vi "(SUBTASK 3) - Read and display material.vi"() -> ()   [LabVIEW 2016, in "testrobot.lvrbt"]
uses:
  testrobot.lvrbt
  <vilib>/NXT/Block Support/NXT_InputPort.ctl
  <vilib>/NXT/Subs/LVHSConnector.ctl
  <vilib>/NXT/LegoClasses/BrickReference/BrickReference.lvclass
panel:
  out "Numeric":dbl
  in  "left light":T1 items=["Port 1", "Port 2", "Port 3", "Port 4"]
  in  "right light":T1=3 items=["Port 1", "Port 2", "Port 3", "Port 4"]
  out "only right":bool
  out "both negative":bool
  out "both positve":bool
  out "Left":bool
  out "Right":bool
  out "Right 2":sgl
  out "Left 2":sgl
  out "NXT/EV3 2":T2
  out "Scaled dif":dbl
  in  "NXT/EV3":T2
  in  "Force":T1=1 items=["Port 1", "Port 2", "Port 3", "Port 4"]
  # "Port 2"
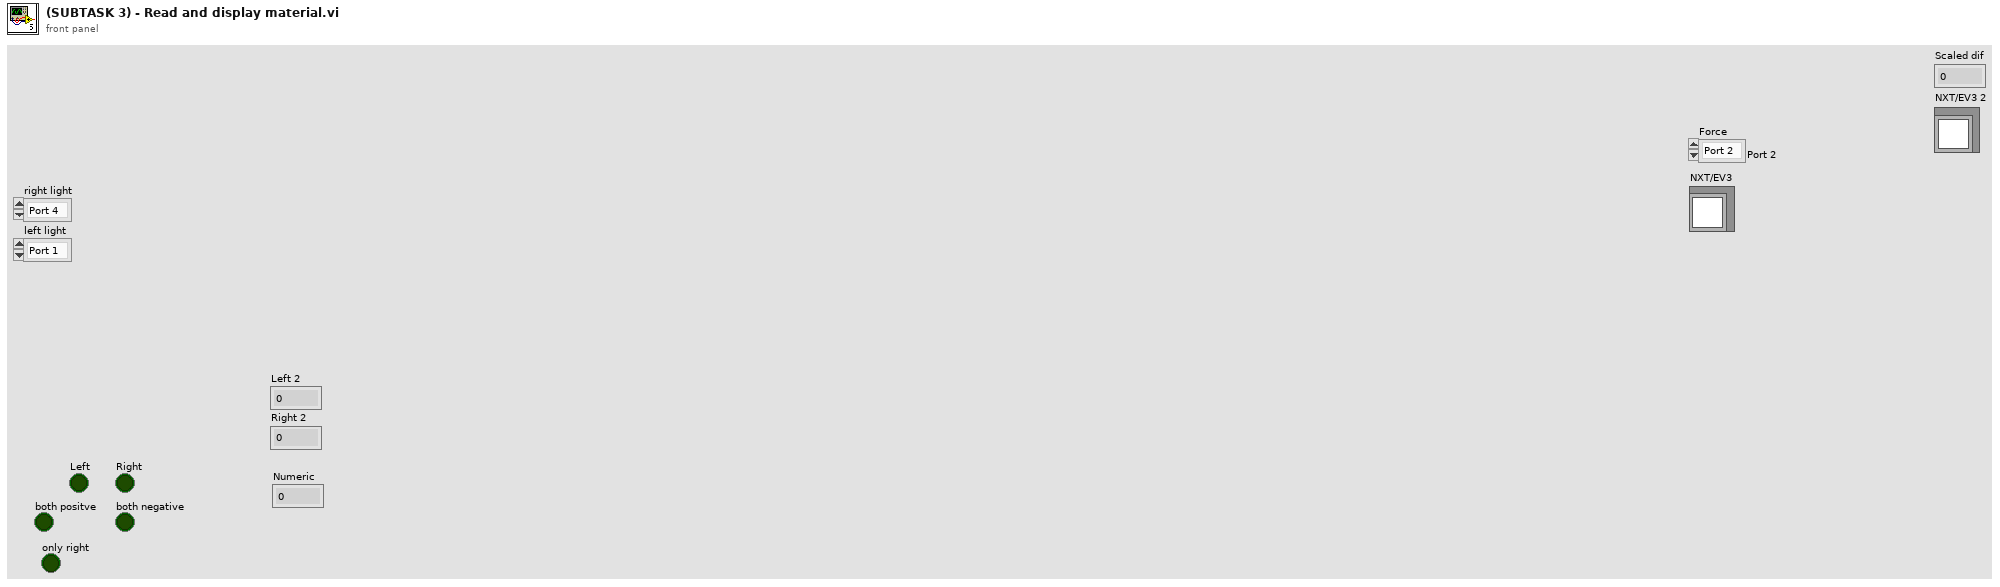
[diagram p1: front panel]
types:
  T1 = typedef "NXT_InputPort.ctl" = u32
  T2 = typedef "LVHSConnector.ctl" = refnum<class "BrickReference.lvclass">
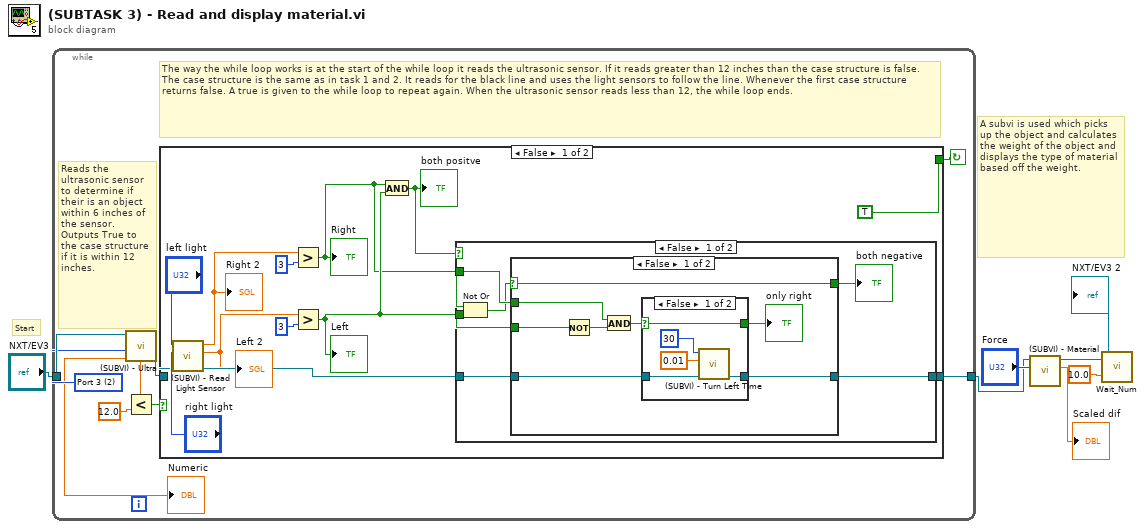
[diagram p0: block diagram]
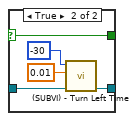
[diagram p2: hidden frame]
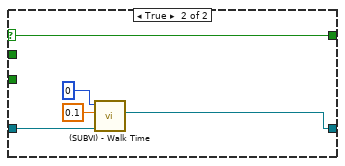
[diagram p3: hidden frame]
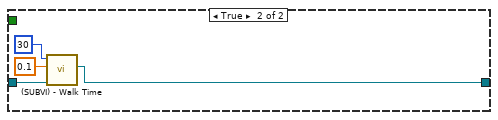
[diagram p4: hidden frame]
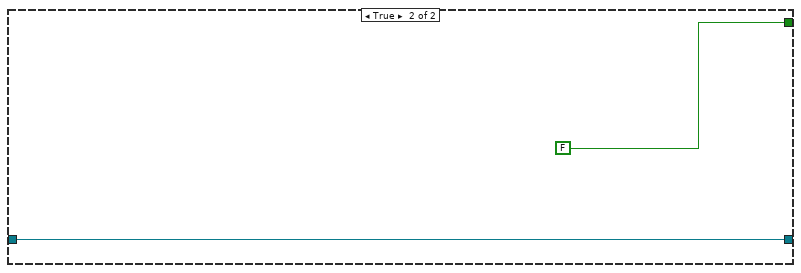
[diagram p5: hidden frame]
diagram:
  # "A subvi is used which picks up the object and calculates the weight of the object and displays the type of material based off the weight."
  # "Start"
  n1 = while {
    tunnel: "NXT/EV3" -> [w15]
    tunnel: [w10] -> w1
    stop <- w12 continue-if-true
    w9 = T1 2 items=["Port 1", "Port 2", "Port 3", "Port 4"] ("Port (Port 1)")
    # "The way the while loop works is at the start of the while loop it reads the ultrasonic sensor. If it reads greater than 12 inches than the case structure is false. The case structure is the same as in task 1 and 2. It reads for the black line and uses the light sensors to follow the line. Whenever the first case structure returns false. A true is given to the while loop to repeat again. When the ultrasonic sensor reads less than 12, the while loop ends."
    # "Reads the ultrasonic sensor to determine if their is an object within 6 inches of the sensor. Outputs True to the case structure if it is within 12 inches."
    n2 = call "(SUBVI) - Ultra.vi"("Port (Port 1)"=w9, "NXT/EV3"=w15) -> ("Inches"=w8:sgl, "NXT/EV3 2"=w11:T2)  [unwired: 8 in]
    "Numeric" <- w8
    n3 = Less?(x=w8, y=sgl 12.0 ("x")) -> (x < y?=w13:bool)
    n4 = case shown="False" w13 {
      tunnel: [TRUE FALSE] -> w12
      tunnel: w11 -> [w18 w62]
      tunnel: [w17 w62] -> w10
      frame False {
        n5 = call "(SUBVI) - Read Light Sensor.vi"("NXT/EV3"=w18, "Port (Port 1) 2"="right light", "Port (Port 1)"="left light") -> ("NXT/EV3 2"=w24:T2, "Scaled Value 2"=w21:sgl, "Scaled Value"=w22:sgl)  [unwired: 6 in]
        "Left 2" <- w21
        "Right 2" <- w22
        n6 = Greater?(x=w22, y=3) -> (0:w25:bool)
        "Right" <- w25
        n7 = Greater?(x=w21, y=3) -> (0:w26:bool)
        "Left" <- w26
        n8 = And(x=w25, y=w26) -> (x .and. y?=w23:bool)
        "both positve" <- w23
        n9 = case shown="False" w23 {
          tunnel: w24 -> [w30 w59]
          tunnel: [w29 w58] -> w17
          tunnel: w25 -> [w33 _]
          tunnel: w26 -> [w32 _]
          frame False {
            n10 = Not Or(1:w32, 2:w33) -> (0:w31:bool)
            n11 = case shown="False" w31 {
              selector: w31 -> [w42 w57]
              tunnel: [w42 w57] -> w34
              tunnel: w33 -> [w40 _]
              tunnel: w32 -> [w38 _]
              tunnel: w30 -> [w36 w54]
              tunnel: [w35 w53] -> w29
              frame False {
                n12 = Not(x=w38) -> (.not. x?=w39:bool)
                n13 = And(x=w40, y=w39) -> (x .and. y?=w41:bool)
                n14 = case shown="False" w41 {
                  selector: w41 -> [w47 w52]
                  tunnel: [w47 w52] -> w37
                  tunnel: w36 -> [w44 w49]
                  tunnel: [w43 w48] -> w35
                  frame False {
                    n15 = call "(SUBVI) - Turn Left Time.vi"("NXT/EV3"=w44, "Time walking"=0.01, "Walk Speed"=30) -> ("NXT/EV3 2"=w43:T2)  [unwired: 8 in]
                  }
                  frame True {
                    n16 = call "(SUBVI) - Turn Left Time.vi"("NXT/EV3"=w49, "Time walking"=0.01, "Walk Speed"=-30) -> ("NXT/EV3 2"=w48:T2)  [unwired: 8 in]
                  }
                }
                "only right" <- w37
              }
              frame True {
                n17 = call "(SUBVI) - Walk Time.vi"("NXT/EV3"=w54, "Time walking"=0.1, "Walk Speed"=0) -> ("NXT/EV3 2"=w53:T2)  [unwired: 8 in]
              }
            }
            "both negative" <- w34
          }
          frame True {
            n18 = call "(SUBVI) - Walk Time.vi"("NXT/EV3"=w59, "Time walking"=0.1, "Walk Speed"=30) -> ("NXT/EV3 2"=w58:T2)  [unwired: 8 in]
          }
        }
      }
      frame True {
      }
    }
  }
  n19 = call "(SUBVI) - Material.vi"("Port (Port 1)"="Force", "NXT/EV3"=w1) -> ("Scaled dif"=→"Scaled dif":dbl, "NXT/EV3 2"=w4:T2)  [unwired: 8 in]
  n20 = call <vilib>:"Wait_Num.vi"("Time (1 sec)"=sgl 10.0, "NXT/EV3"=w4) -> ("NXT/EV3"=→"NXT/EV3 2":T2)  [unwired: 2 in]
